vi "Update Parameters Values.vi"(8 "error in":errorcluster, 9 "message fields":T1 {"data" format="%x"; "extra" format="%x"; "msgopt" format="%04x"; "msgflag" format="%04x"; "bus" items=["BUSA", "BUSB", "BUSNONE"]; "cwd1" format="%04x"; "cwd2" format="%04x"; "swd1" format="%04x"; "swd2" format="%04x"}, 10 "values in":dbl[](array[numeric]), 11 "Rx execution unit in":refnum<class "Rx Execution Unit.lvclass">) -> (0 "error out":errorcluster, 1 "status error counts":T2, 2 "values out":dbl[](array[numeric]), 3 "Rx execution unit out":refnum<class "Rx Execution Unit.lvclass">)   [LabVIEW 2020, in "AIM MIL-STD-1553 Engine.lvlib" / "Implementation.lvlib" / "Rx Execution Unit.lvclass"]
uses:
  Rx Execution Unit.lvclass
  Status Error Counts.ctl
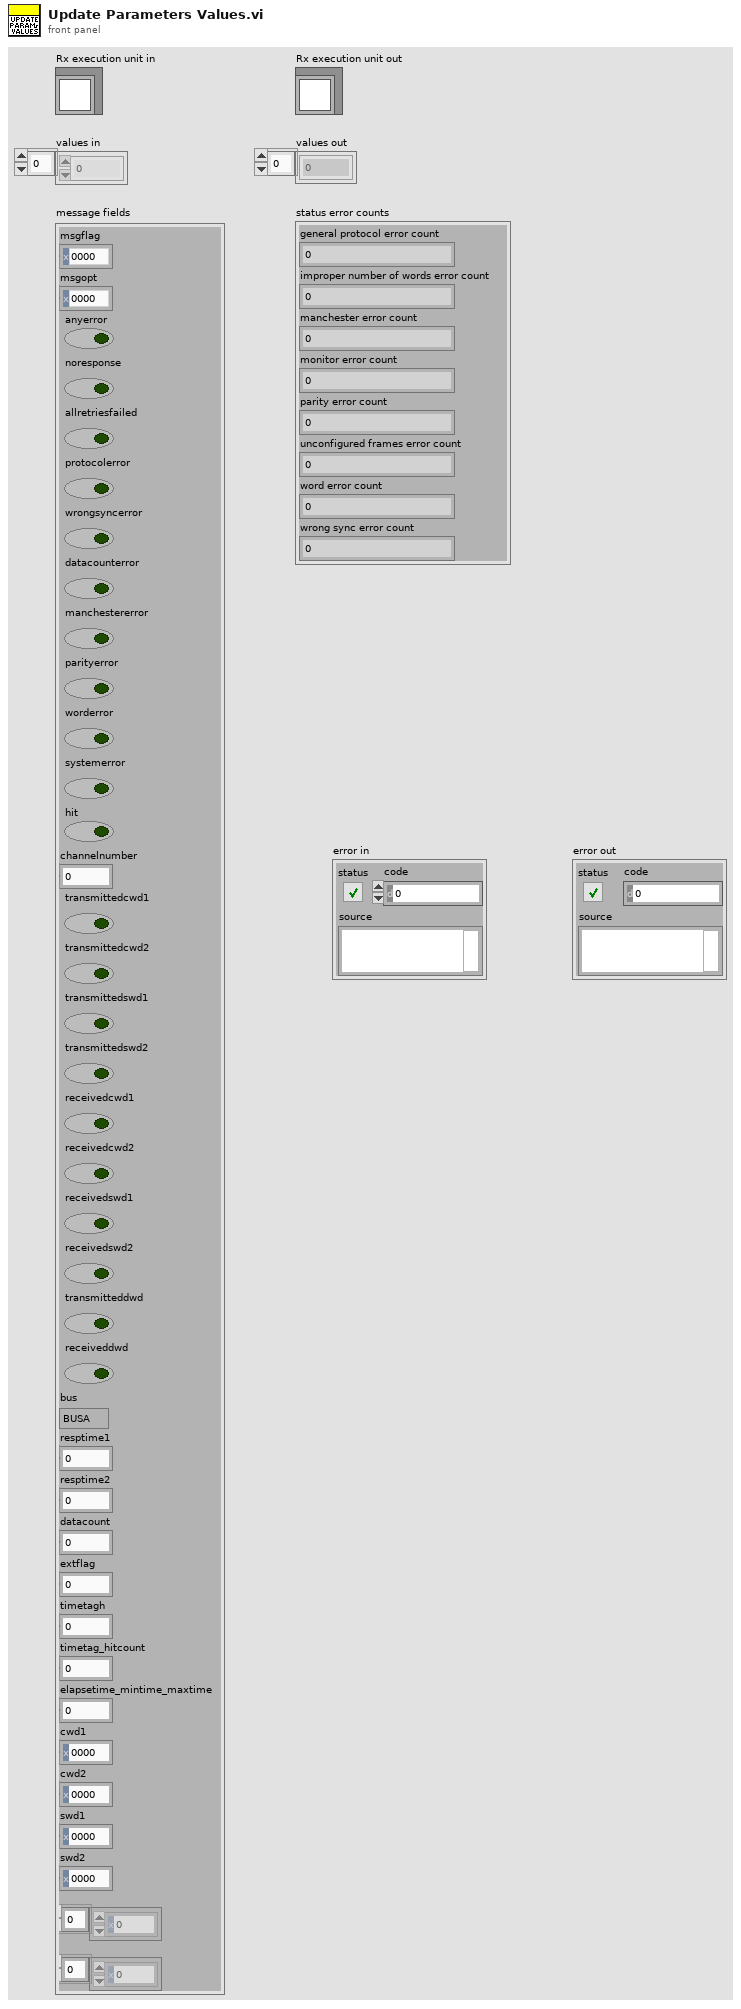
[diagram p1: front panel]
types:
  T1 = cluster{"msgflag":u16, "msgopt":u16, "anyerror":bool, "noresponse":bool, "allretriesfailed":bool, "protocolerror":bool, "wrongsyncerror":bool, "datacounterror":bool, "manchestererror":bool, "parityerror":bool, "worderror":bool, "systemerror":bool, "hit":bool, "reserved":u8, "channelnumber":i32, "transmittedcwd1":bool, "transmittedcwd2":bool, "transmittedswd1":bool, "transmittedswd2":bool, "receivedcwd1":bool, "receivedcwd2":bool, "receivedswd1":bool, "receivedswd2":bool, "transmitteddwd":bool, "receiveddwd":bool, "reserved":i8, "reserved":i8, "bus":u32, "resptime1":u16, "resptime2":u16, "datacount":u16, "extflag":u16, "timetagh":u32, "timetag_hitcount":u32, "elapsetime_mintime_maxtime":u32, "cwd1":u16, "cwd2":u16, "swd1":u16, "swd2":u16, "data":u16[], "extra":u16[]}
  T2 = typedef "AIM MIL-STD-1553 Engine.lvlib/Implementation.lvlib/Rx Execution Unit.lvclass/Status Error Counts.ctl" = cluster{"general protocol error count":u64, "improper number of words error count":u64, "manchester error count":u64, "monitor error count":u64, "parity error count":u64, "unconfigured frames error count":u64, "word error count":u64, "wrong sync error count":u64}
  T3 = typedef "Map of Messages to Value Indexes.ctl" = map{T4, T5}
  T4 = typedef "Message Map Key.ctl" = cluster{"HW channel":u16, "terminal address":u16, "subaddress":u16, "mode code":u16}
  T5 = typedef "AIM MIL-STD-1553 Engine.lvlib/Implementation.lvlib/Rx Execution Unit.lvclass/Message Map Value.ctl" = cluster{"value indexes":i32[], "message":T6, "Tx status count":i32, "Rx status count":i32}
  T6 = typedef "Message Definition.ctl" = cluster{"name":string, "message type":T7, "endpoint Tx":T8, "endpoint Rx":T8, "create timestamp channel":bool, "mode code":u16, "number of words":u16, "parameters":cluster{"name":string, "default value":dbl, "unit":string, "parameter definition":T10}[]}
  T7 = typedef "Message Type.ctl" = string
  T8 = typedef "Terminal Endpoint.ctl" = cluster{"terminal address":T9, "subaddress":T9}
  T9 = typedef "Address.ctl" = u16
  T10 = typedef "Parameter Definition.ctl" = cluster{"start index":i32, "size (bits)":i32, "encoding":enum16{"BNR", "BCD", "Discrete"}, "signed":bool, "multiplier":dbl, "offset":dbl}
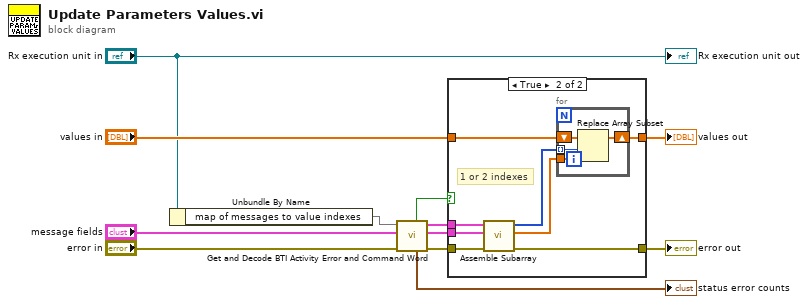
[diagram p0: block diagram]
diagram:
  n1 = Unbundle By Name("Rx execution unit in") -> ("map of messages to value indexes"=w12:T3)
  n2 = call "Get and Decode BTI Activity Error and Command Word.vi"("error in"="error in", "message fields"="message fields", "map of messages to value indexes"=w12) -> ("error out"=w5:errorcluster, "message fields out"=w9:T1, "value"=w8:T5, "status error counts"=→"status error counts":T2, "update values"=w10:bool)  [unwired: 4 in]
  n3 = case shown="True" w10 {
    tunnel: "values in" -> [w14 w22]
    tunnel: w5 -> [w13 w16]
    tunnel: [w13 w21] -> w4
    tunnel: [w14 w20] -> w6
    tunnel: w8 -> [_ w17]
    tunnel: w9 -> [_ w15]
    frame False {
    }
    frame True {
      # "1 or 2 indexes"
      n4 = call "Assemble Subarray.vi"("error in"=w16, "message fields"=w15, "message"=w17) -> ("error out"=w21:errorcluster, "subarray"=w18:dbl[], "value indexes"=w19:i32[])  [unwired: 6 in]
      n5 = for {
        shift-right: [w26] -> w20
        shift-left: w22 -> [w25]
        tunnel: w19 -> [w24] mode=indexing
        tunnel: w18 -> [w23]
        # "For Each value index"
        n6 = Replace Array Subset(array=w25, new element=w23, index=w24) -> (w26:dbl[])
      }
    }
  }
  "values out" <- w6
  "error out" <- w4
  "Rx execution unit out" <- "Rx execution unit in"
